vi "qalibrate.vi"() -> ()   [LabVIEW 2019, in "Global.lvlib"]
uses:
  Global.lvlib
panel:
  in  "RunFromCalibrate":bool
  in  "Status":string="0"
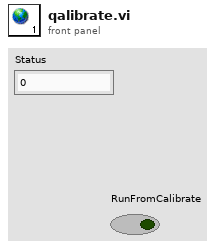
[diagram p1: front panel]
diagram:
